vi "constants_LL.vi"(8 "NumKneeMotorsInUse":i32, 9 "NumPelvisMotorsInUse":i32, 10 "MotorsInUse":bool[](array[boolean])=[FALSE, FALSE, FALSE, FALSE, FALSE, FALSE, FALSE, FALSE], 11 "NumTrunkMotorsInUse":i32) -> (3 "Constants LL":T1)   [LabVIEW 2024]
uses:
  typeDef/constants_LL.ctl
panel:
  in  "Constants LL 2":T1
  out "whichMotors":i32[](array[numeric])
  out "nMotors":i32
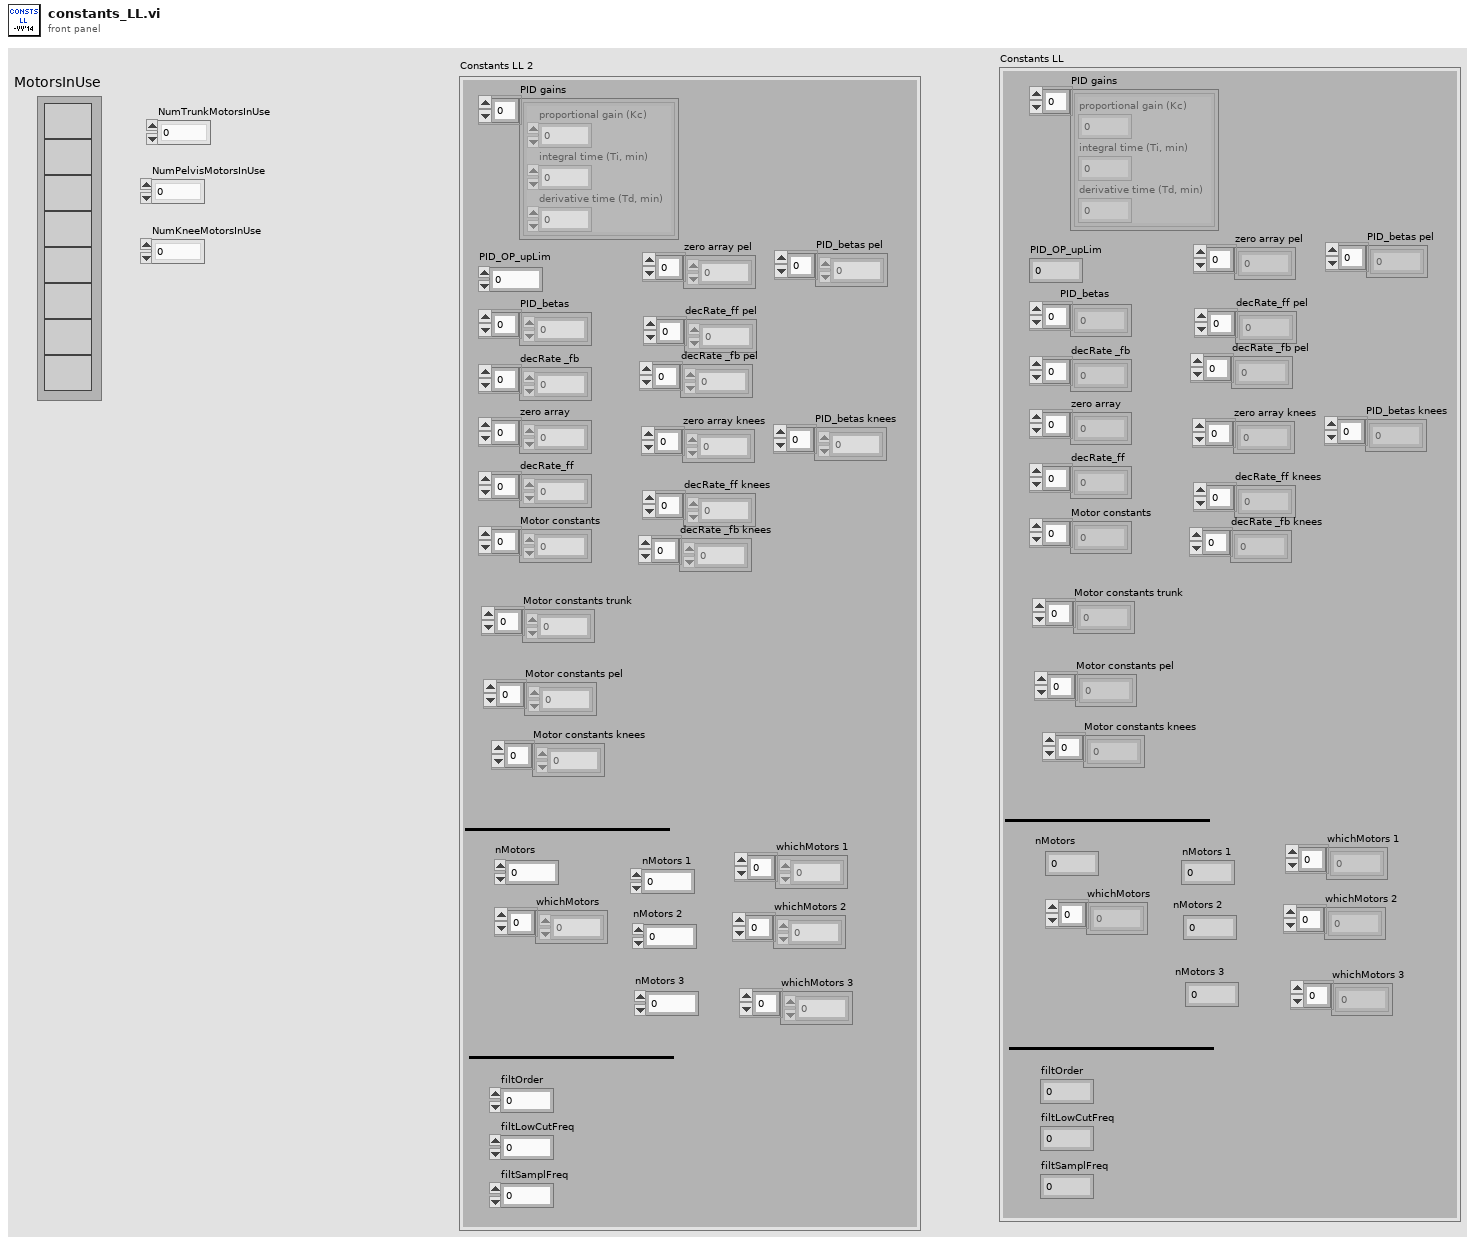
[diagram p1: front panel]
types:
  T1 = typedef "constants_LL.ctl" = cluster{"zero array":dbl[], "decRate_ff":dbl[], "Motor constants":dbl[], "PID gains":cluster{"proportional gain (Kc)":dbl, "integral time (Ti, min)":dbl, "derivative time (Td, min)":dbl}[], "decRate _fb":dbl[], "PID_OP_upLim":dbl, "nMotors":i32, "PID_betas":dbl[], "filtOrder":i32, "filtLowCutFreq":dbl, "filtSamplFreq":dbl, "whichMotors":i32[], "nMotors 1":i32, "nMotors 2":i32, "Motor constants pel":dbl[], "Motor constants trunk":dbl[], "whichMotors 1":i32[], "whichMotors 2":i32[], "zero array pel":dbl[], "decRate_ff pel":dbl[], "decRate _fb pel":dbl[], "PID_betas pel":dbl[], "whichMotors 3":i32[], "nMotors 3":i32, "Motor constants knees":dbl[], "zero array knees":dbl[], "decRate_ff knees":dbl[], "decRate _fb knees":dbl[], "PID_betas knees":dbl[]}
  T2 = cluster{"proportional gain (Kc)":dbl, "integral time (Ti, min)":dbl, "derivative time (Td, min)":dbl}[]
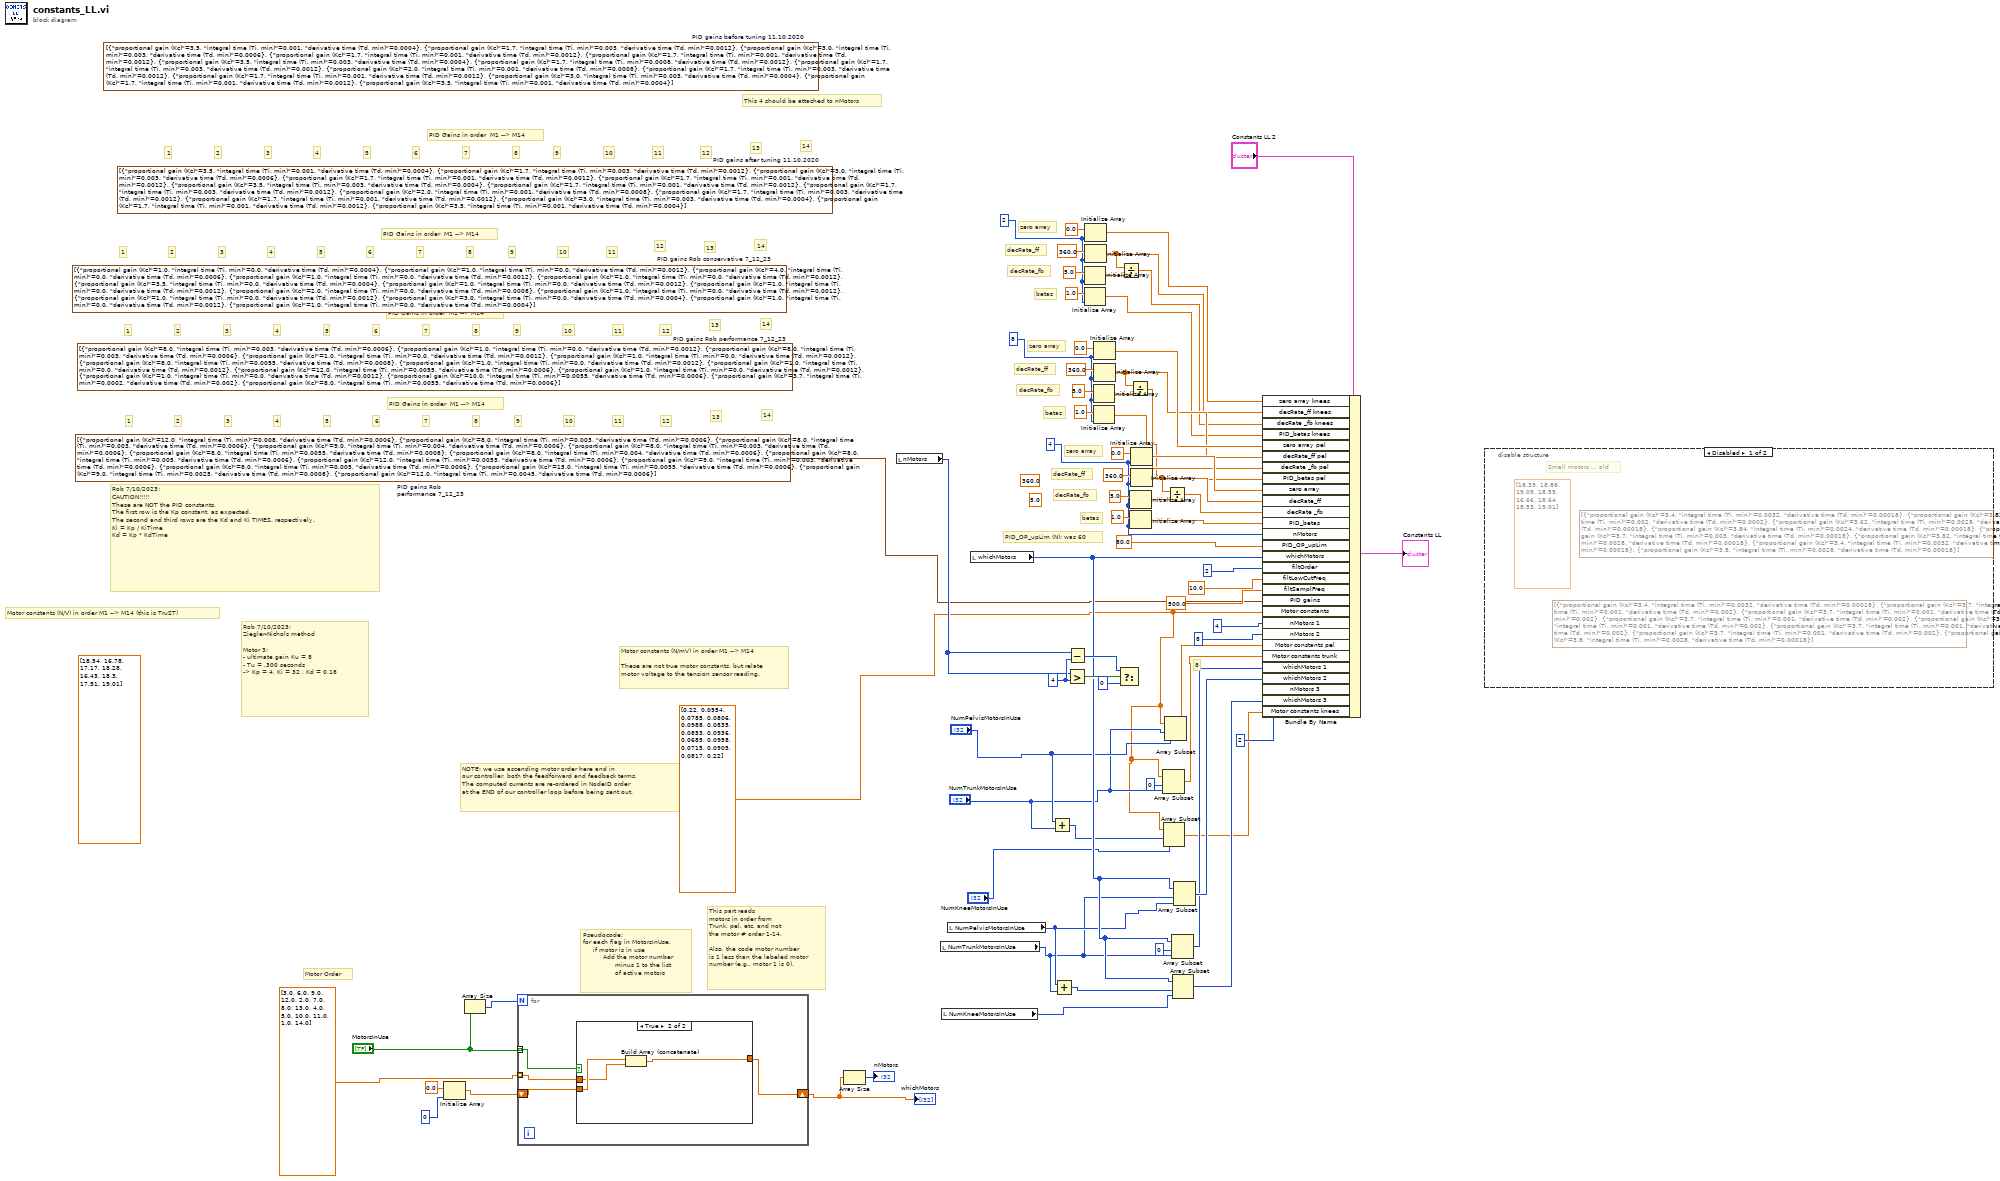
[diagram p0: block diagram]
diagram:
  (unwired) T2 [{"proportional gain (Kc)"=8.0, "integral time (Ti, min)"=0.003, "derivative time (Td, min)"=0.0006}, {"proportional gain (Kc)"=1.0, "integral time (Ti, min)"=0.0, "derivative time (Td, min)"=0.0012}, {"proportional gain (Kc)"=8.0, "integral time (Ti, min)"=0.003, "derivative time (Td, min)"=0.0006}, {"proportional gain (Kc)"=1.0, "integral time (Ti, min)"=0.0, "derivative time (Td, min)"=0.0012}, {"proportional gain (Kc)"=1.0, "integral time (Ti, min)"=0.0, "derivative time (Td, min)"=0.0012}, {"proportional gain (Kc)"=8.0, "integral time (Ti, min)"=0.0055, "derivative time (Td, min)"=0.0008}, {"proportional gain (Kc)"=1.0, "integral time (Ti, min)"=0.0, "derivative time (Td, min)"=0.0012}, {"proportional gain (Kc)"=1.0, "integral time (Ti, min)"=0.0, "derivative time (Td, min)"=0.0012}, {"proportional gain (Kc)"=12.0, "integral time (Ti, min)"=0.0055, "derivative time (Td, min)"=0.0006}, {"proportional gain (Kc)"=1.0, "integral time (Ti, min)"=0.0, "derivative time (Td, min)"=0.0012}, {"proportional gain (Kc)"=1.0, "integral time (Ti, min)"=0.0, "derivative time (Td, min)"=0.0012}, {"proportional gain (Kc)"=10.0, "integral time (Ti, min)"=0.0055, "derivative time (Td, min)"=0.0006}, {"proportional gain (Kc)"=3.7, "integral time (Ti, min)"=0.0002, "derivative time (Td, min)"=0.002}, {"proportional gain (Kc)"=8.0, "integral time (Ti, min)"=0.0055, "derivative time (Td, min)"=0.0006}]  # PID gains Rob performance 7_12_23
  w9 = T2 [{"proportional gain (Kc)"=12.0, "integral time (Ti, min)"=0.008, "derivative time (Td, min)"=0.0006}, {"proportional gain (Kc)"=8.0, "integral time (Ti, min)"=0.003, "derivative time (Td, min)"=0.0006}, {"proportional gain (Kc)"=8.0, "integral time (Ti, min)"=0.003, "derivative time (Td, min)"=0.0006}, {"proportional gain (Kc)"=9.0, "integral time (Ti, min)"=0.004, "derivative time (Td, min)"=0.0006}, {"proportional gain (Kc)"=8.0, "integral time (Ti, min)"=0.003, "derivative time (Td, min)"=0.0006}, {"proportional gain (Kc)"=8.0, "integral time (Ti, min)"=0.0055, "derivative time (Td, min)"=0.0008}, {"proportional gain (Kc)"=8.0, "integral time (Ti, min)"=0.004, "derivative time (Td, min)"=0.0006}, {"proportional gain (Kc)"=8.0, "integral time (Ti, min)"=0.005, "derivative time (Td, min)"=0.0006}, {"proportional gain (Kc)"=12.0, "integral time (Ti, min)"=0.0055, "derivative time (Td, min)"=0.0006}, {"proportional gain (Kc)"=9.0, "integral time (Ti, min)"=0.003, "derivative time (Td, min)"=0.0006}, {"proportional gain (Kc)"=8.0, "integral time (Ti, min)"=0.005, "derivative time (Td, min)"=0.0006}, {"proportional gain (Kc)"=15.0, "integral time (Ti, min)"=0.0055, "derivative time (Td, min)"=0.0006}, {"proportional gain (Kc)"=9.0, "integral time (Ti, min)"=0.0025, "derivative time (Td, min)"=0.0008}, {"proportional gain (Kc)"=12.0, "integral time (Ti, min)"=0.0045, "derivative time (Td, min)"=0.0006}]  # PID gains Rob performance 7_12_23
  (unwired) T2 [{"proportional gain (Kc)"=1.0, "integral time (Ti, min)"=0.0, "derivative time (Td, min)"=0.0004}, {"proportional gain (Kc)"=1.0, "integral time (Ti, min)"=0.0, "derivative time (Td, min)"=0.0012}, {"proportional gain (Kc)"=4.0, "integral time (Ti, min)"=0.0, "derivative time (Td, min)"=0.0006}, {"proportional gain (Kc)"=1.0, "integral time (Ti, min)"=0.0, "derivative time (Td, min)"=0.0012}, {"proportional gain (Kc)"=1.0, "integral time (Ti, min)"=0.0, "derivative time (Td, min)"=0.0012}, {"proportional gain (Kc)"=3.5, "integral time (Ti, min)"=0.0, "derivative time (Td, min)"=0.0004}, {"proportional gain (Kc)"=1.0, "integral time (Ti, min)"=0.0, "derivative time (Td, min)"=0.0012}, {"proportional gain (Kc)"=1.0, "integral time (Ti, min)"=0.0, "derivative time (Td, min)"=0.0012}, {"proportional gain (Kc)"=2.0, "integral time (Ti, min)"=0.0, "derivative time (Td, min)"=0.0008}, {"proportional gain (Kc)"=1.0, "integral time (Ti, min)"=0.0, "derivative time (Td, min)"=0.0012}, {"proportional gain (Kc)"=1.0, "integral time (Ti, min)"=0.0, "derivative time (Td, min)"=0.0012}, {"proportional gain (Kc)"=3.0, "integral time (Ti, min)"=0.0, "derivative time (Td, min)"=0.0004}, {"proportional gain (Kc)"=1.0, "integral time (Ti, min)"=0.0, "derivative time (Td, min)"=0.0012}, {"proportional gain (Kc)"=1.0, "integral time (Ti, min)"=0.0, "derivative time (Td, min)"=0.0004}]  # PID gains Rob conservative 7_12_23
  (unwired) T2 [{"proportional gain (Kc)"=3.5, "integral time (Ti, min)"=0.001, "derivative time (Td, min)"=0.0004}, {"proportional gain (Kc)"=1.7, "integral time (Ti, min)"=0.003, "derivative time (Td, min)"=0.0012}, {"proportional gain (Kc)"=3.0, "integral time (Ti, min)"=0.003, "derivative time (Td, min)"=0.0006}, {"proportional gain (Kc)"=1.7, "integral time (Ti, min)"=0.001, "derivative time (Td, min)"=0.0012}, {"proportional gain (Kc)"=1.7, "integral time (Ti, min)"=0.001, "derivative time (Td, min)"=0.0012}, {"proportional gain (Kc)"=3.5, "integral time (Ti, min)"=0.003, "derivative time (Td, min)"=0.0004}, {"proportional gain (Kc)"=1.7, "integral time (Ti, min)"=0.0008, "derivative time (Td, min)"=0.0012}, {"proportional gain (Kc)"=1.7, "integral time (Ti, min)"=0.003, "derivative time (Td, min)"=0.0012}, {"proportional gain (Kc)"=2.0, "integral time (Ti, min)"=0.001, "derivative time (Td, min)"=0.0008}, {"proportional gain (Kc)"=1.7, "integral time (Ti, min)"=0.003, "derivative time (Td, min)"=0.0012}, {"proportional gain (Kc)"=1.7, "integral time (Ti, min)"=0.001, "derivative time (Td, min)"=0.0012}, {"proportional gain (Kc)"=3.0, "integral time (Ti, min)"=0.003, "derivative time (Td, min)"=0.0004}, {"proportional gain (Kc)"=1.7, "integral time (Ti, min)"=0.001, "derivative time (Td, min)"=0.0012}, {"proportional gain (Kc)"=3.5, "integral time (Ti, min)"=0.001, "derivative time (Td, min)"=0.0004}]  # PID gains before tuning 11.10.2020
  (unwired) T2 [{"proportional gain (Kc)"=3.5, "integral time (Ti, min)"=0.001, "derivative time (Td, min)"=0.0004}, {"proportional gain (Kc)"=1.7, "integral time (Ti, min)"=0.003, "derivative time (Td, min)"=0.0012}, {"proportional gain (Kc)"=3.0, "integral time (Ti, min)"=0.003, "derivative time (Td, min)"=0.0006}, {"proportional gain (Kc)"=1.7, "integral time (Ti, min)"=0.001, "derivative time (Td, min)"=0.0012}, {"proportional gain (Kc)"=1.7, "integral time (Ti, min)"=0.001, "derivative time (Td, min)"=0.0012}, {"proportional gain (Kc)"=3.5, "integral time (Ti, min)"=0.003, "derivative time (Td, min)"=0.0004}, {"proportional gain (Kc)"=1.7, "integral time (Ti, min)"=0.001, "derivative time (Td, min)"=0.0012}, {"proportional gain (Kc)"=1.7, "integral time (Ti, min)"=0.003, "derivative time (Td, min)"=0.0012}, {"proportional gain (Kc)"=2.0, "integral time (Ti, min)"=0.001, "derivative time (Td, min)"=0.0008}, {"proportional gain (Kc)"=1.7, "integral time (Ti, min)"=0.003, "derivative time (Td, min)"=0.0012}, {"proportional gain (Kc)"=1.7, "integral time (Ti, min)"=0.001, "derivative time (Td, min)"=0.0012}, {"proportional gain (Kc)"=3.0, "integral time (Ti, min)"=0.003, "derivative time (Td, min)"=0.0004}, {"proportional gain (Kc)"=1.7, "integral time (Ti, min)"=0.001, "derivative time (Td, min)"=0.0012}, {"proportional gain (Kc)"=3.5, "integral time (Ti, min)"=0.001, "derivative time (Td, min)"=0.0004}]  # PID gains after tuning 11.10.2020
  w27 = 2 ("nMotors")
  w37 = 8 ("nMotors")
  w46 = 4 ("nMotors")
  (unwired) 5.0 ("element")
  (unwired) 360.0 ("element")
  w53 = 4 ("y")
  w8 = dbl[] [0.22, 0.0954, 0.0785, 0.0806, 0.0988, 0.0835, 0.0853, 0.0936, 0.0685, 0.0958, 0.0715, 0.0905, 0.0817, 0.22]
  (unwired) dbl[] [18.54, 16.78, 17.17, 18.28, 16.43, 18.3, 17.51, 19.01]
  # "14"
  # "13"
  # "12"
  # "11"
  # "10"
  # "9"
  # "8"
  # "7"
  # "6"
  # "5"
  # "4"
  # "3"
  # "1"
  # "2"
  # "PID Gains in order  M1 --> M14"
  # "Pseudocode: \nfor each flag in MotorsInUse, \n     if motor is in use\n          Add the motor number \n                minus 1 to the list\n                of active motors"
  # "14"
  # "13"
  # "12"
  # "11"
  # "10"
  # "9"
  # "8"
  # "7"
  # "6"
  # "5"
  # "4"
  # "3"
  # "1"
  # "2"
  # "PID Gains in order  M1 --> M14"
  # "Rob 7/10/2023: \nCAUTION!!!!!\nThese are NOT the PID constants. \nThe first row is the Kp constant, as expected. \nThe second and third rows are the Kd and Ki TIMES, respectively. \nKi = Kp / KiTime\nKd = Kp * KdTime"
  # "NOTE: we use ascending motor order here and in\nour controller, both the feedforward and feedback terms. \nThe computed currents are re-ordered in NodeID order \nat the END of our controller loop before being sent out."
  # "Rob 7/10/2023: \nZiegler-Nichols method\n\nMotor 3: \n- ultimate gain Ku = 8\n- Tu = .300 seconds\n-> Kp = 4, Ki = 32 , Kd = 0.18"
  # "14"
  # "13"
  # "12"
  # "11"
  # "10"
  # "9"
  # "8"
  # "7"
  # "6"
  # "5"
  # "4"
  # "3"
  # "1"
  # "2"
  # "PID Gains in order  M1 --> M14"
  # "14"
  # "13"
  # "12"
  # "11"
  # "10"
  # "9"
  # "8"
  # "7"
  # "6"
  # "5"
  # "4"
  # "3"
  # "1"
  # "2"
  # "decRate_fb"
  # "decRate_ff"
  # "zero array"
  # "betas"
  # "8"
  # "decRate_fb"
  # "decRate_ff"
  # "zero array"
  # "betas"
  # "This 4 should be attached to nMotors"
  # "This part reads\nmotors in order from\nTrunk, pel, etc, and not\nthe motor # order 1-14. \n\nAlso, the code motor number\nis 1 less than the labeled motor \nnumber (e.g., motor 1 is 0)."
  # "Motor Order"
  # "Motor constants (N/mV) in order M1 --> M14\n\nThese are not true motor constants, but relate\nmotor voltage to the tension sensor reading."
  # "decRate_fb"
  # "decRate_ff"
  # "zero array"
  # "betas"
  # "PID_OP_upLim (N): was 60"
  # "PID Gains in order  M1 --> M14"
  # "Motor constants (N/V) in order M1 --> M14 (this is TruST)"
  n1 = Initialize Array(0.0 ("element"), 0 ("dimension size")) -> (w3:dbl[])
  n2 = Array Size(array="MotorsInUse") -> (size(s)=w7:i32)
  n3 = for {
    N: w7 -> [_]
    tunnel: "MotorsInUse" -> [w75] mode=indexing
    shift-right: [w73] -> w1
    shift-left: w3 -> [w74]
    tunnel: dbl[] [3.0, 6.0, 9.0, 12.0, 2.0, 7.0, 8.0, 13.0, 4.0, 5.0, 10.0, 11.0, 1.0, 14.0] -> [w72] mode=indexing
    n4 = case shown="True" w75 {
      tunnel: w74 -> [w76 w79]
      tunnel: [w76 w78] -> w73
      tunnel: w72 -> [_ w77]
      frame False {
      }
      frame True {
        n5 = Build Array (concatenate)(w79, w77) -> (w78:dbl[])
      }
    }
  }
  "whichMotors" <- w1
  n6 = Array Size(array=w1) -> (size(s)=→"nMotors":i32)
  n7 = local read "nMotors"() -> (w47:i32)
  n8 = local read "NumTrunkMotorsInUse"() -> (w11:i32)
  n9 = local read "NumKneeMotorsInUse"() -> (w16:i32)
  n10 = local read "NumPelvisMotorsInUse"() -> (w12:i32)
  n11 = local read "whichMotors"() -> (w22:i32[])
  n12 = Add(x="NumPelvisMotorsInUse", y="NumTrunkMotorsInUse") -> (x+y=w13:i32)
  n13 = Add(x=w12, y=w11) -> (x+y=w10:i32)
  n14 = Greater?(x=w47, y=w53) -> (0:w55:bool)
  n15 = Subtract(x=w47, y=w53) -> (x-y=w54:i32)
  n16 = Initialize Array(5.0 ("element"), w27) -> (w31:dbl[])
  n17 = Initialize Array(1.0 ("element"), w27) -> (w23:dbl[])
  n18 = Initialize Array(0.0 ("element"), w27) -> (w26:dbl[])
  n19 = Initialize Array(360.0 ("element"), w27) -> (w25:dbl[])
  n20 = Initialize Array(5.0 ("element"), w37) -> (w41:dbl[])
  n21 = Initialize Array(1.0 ("element"), w37) -> (w33:dbl[])
  n22 = Initialize Array(0.0 ("element"), w37) -> (w36:dbl[])
  n23 = Initialize Array(360.0 ("element"), w37) -> (w35:dbl[])
  n24 = Select(t=w54, s=w55, f=0) -> ()  [unwired: 1 out]
  n25 = Divide(x=w25, y=w31) -> (x/y=w24:dbl[])
  n26 = Divide(x=w35, y=w41) -> (x/y=w34:dbl[])
  n27 = Initialize Array(5.0 ("element"), w46) -> (w69:dbl[])
  n28 = Initialize Array(1.0 ("element"), w46) -> (w61:dbl[])
  n29 = Initialize Array(0.0 ("element"), w46) -> (w70:dbl[])
  n30 = Initialize Array(360.0 ("element"), w46) -> (w68:dbl[])
  n31 = Array Subset(array=w8, index=0, length="NumTrunkMotorsInUse") -> (w48:dbl[])
  n32 = Array Subset(array=w8, index=w13, length="NumKneeMotorsInUse") -> (w19:dbl[])
  n33 = Array Subset(array=w8, index="NumTrunkMotorsInUse", length="NumPelvisMotorsInUse") -> (w50:dbl[])
  n34 = Divide(x=w68, y=w69) -> (x/y=w67:dbl[])
  n35 = Array Subset(array=w22, index=0, length=w11) -> (w43:i32[])
  n36 = Array Subset(array=w22, index=w10, length=w16) -> (w21:i32[])
  n37 = Array Subset(array=w22, index=w11, length=w12) -> (w44:i32[])
  n38 = Bundle By Name(cluster="Constants LL 2", "zero array knees"=w26, "decRate_ff knees"=w25, "decRate _fb knees"=w24, "PID_betas knees"=w23, "zero array pel"=w36, "decRate_ff pel"=w35, "decRate _fb pel"=w34, "PID_betas pel"=w33, "zero array"=w70, "decRate_ff"=w68, "decRate _fb"=w67, "PID_betas"=w61, "nMotors"=w46, "PID_OP_upLim"=80.0, "whichMotors"=w22, "filtOrder"=2 ("order"), "filtLowCutFreq"=10.0 ("low cutoff freq: fl"), "filtSamplFreq"=500.0 ("sampling freq: fs"), "PID gains"=w9, "Motor constants"=w8, "nMotors 1"=4, "nMotors 2"=8, "Motor constants pel"=w50, "Motor constants trunk"=w48, "whichMotors 1"=w43, "whichMotors 2"=w44, "nMotors 3"=2, "whichMotors 3"=w21, "Motor constants knees"=w19) -> (→"Constants LL":T1)
  n39 = disable-structure shown="Disabled" {
    frame Disabled {
      (unwired) T2 [{"proportional gain (Kc)"=3.4, "integral time (Ti, min)"=0.0032, "derivative time (Td, min)"=0.00018}, {"proportional gain (Kc)"=3.7, "integral time (Ti, min)"=0.001, "derivative time (Td, min)"=0.002}, {"proportional gain (Kc)"=3.7, "integral time (Ti, min)"=0.001, "derivative time (Td, min)"=0.002}, {"proportional gain (Kc)"=3.7, "integral time (Ti, min)"=0.001, "derivative time (Td, min)"=0.002}, {"proportional gain (Kc)"=3.7, "integral time (Ti, min)"=0.001, "derivative time (Td, min)"=0.002}, {"proportional gain (Kc)"=3.7, "integral time (Ti, min)"=0.001, "derivative time (Td, min)"=0.002}, {"proportional gain (Kc)"=3.7, "integral time (Ti, min)"=0.001, "derivative time (Td, min)"=0.002}, {"proportional gain (Kc)"=3.8, "integral time (Ti, min)"=0.0028, "derivative time (Td, min)"=0.00018}] ("PID gains")
      (unwired) T2 [{"proportional gain (Kc)"=3.4, "integral time (Ti, min)"=0.0032, "derivative time (Td, min)"=0.00018}, {"proportional gain (Kc)"=3.82, "integral time (Ti, min)"=0.002, "derivative time (Td, min)"=0.0002}, {"proportional gain (Kc)"=3.62, "integral time (Ti, min)"=0.0028, "derivative time (Td, min)"=0.00018}, {"proportional gain (Kc)"=3.84, "integral time (Ti, min)"=0.0024, "derivative time (Td, min)"=0.00018}, {"proportional gain (Kc)"=3.7, "integral time (Ti, min)"=0.003, "derivative time (Td, min)"=0.00018}, {"proportional gain (Kc)"=3.82, "integral time (Ti, min)"=0.0028, "derivative time (Td, min)"=0.00018}, {"proportional gain (Kc)"=3.4, "integral time (Ti, min)"=0.0032, "derivative time (Td, min)"=0.00018}, {"proportional gain (Kc)"=3.8, "integral time (Ti, min)"=0.0028, "derivative time (Td, min)"=0.00018}] ("PID gains")
      (unwired) dbl[] [18.39, 18.88, 19.09, 18.59, 16.66, 18.64, 18.53, 19.01]
      # "Small motors ... old"
    }
    frame Enabled {
    }
  }
